vi "CMD - shutdown.vi"(8 "error in (no error)":errorcluster, 10 "timeout (ms)":i32=10000, 11 "TipPanelHandle":refnum<class "TipPanelHandle.lvclass">) -> (0 "error out":errorcluster)   [LabVIEW 2021, in "TipStripOOPanel.lvlib" / "TipPanelHandle.lvclass"]
uses:
  TipPanelHandle.lvclass
  TipPanelHandle.lvclass/TipPanelHandle.ctl
  <vilib>/Futures/Futures/Futures.lvlib
  <vilib>/Futures/Futures/Future/Future.lvclass
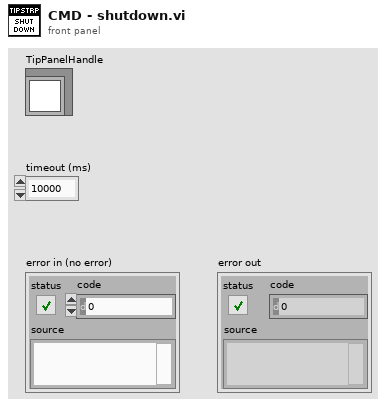
[diagram p1: front panel]
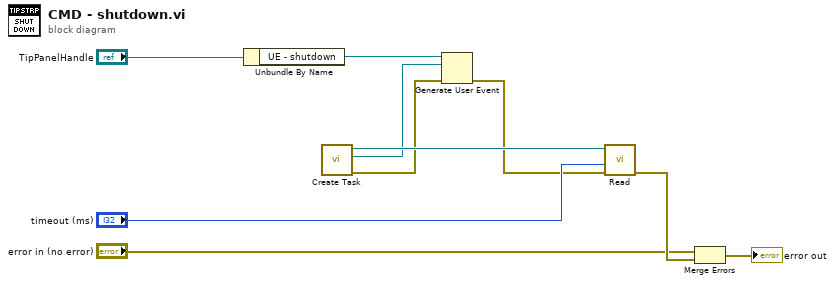
[diagram p0: block diagram]
diagram:
  n1 = Unbundle By Name("TipPanelHandle") -> ("UE - shutdown"=w9:refnum<user-event>)
  n2 = call <vilib>:"Create Task.vi"() -> ("error out"=w5:errorcluster, "Promise out"=w6:refnum<class "Promise.lvclass">, "Future out"=w8:refnum<class "Future.lvclass">)  [unwired: 9 in]
  n3 = Generate User Event(user event=w9, event data cluster=w6, error in=w5) -> (error out=w4:errorcluster)  [unwired: 1 in, 1 out]
  n4 = call <vilib>:"Read.vi"("error in (no error)"=w4, "timeout in ms (60 sec)"="timeout (ms)", "Future in"=w8) -> ("error out"=w3:errorcluster)  [unwired: 5 in, 3 out]
  n5 = Merge Errors("error in (no error)", w3) -> (→"error out":errorcluster)
